vi "sirah.vi"(5 "lower limit":dbl=720.0 format="%#_13g", 6 "resonator_motor, f(x)":string="-2.10126553E+01 * x^2  + 6.31242686E+03 * x + 6.95582109E+05", 7 "upper limit":dbl=690.0 format="%#_13g", 8 "error in (no error)":errorcluster, 10 "wavelength (nm)":dbl=711.0001 format="%#_16g") -> (0 "error out":errorcluster, 1 "fundamental (nm)":dbl=708.9981708820242 format="%.4f", 2 "value out":dbl=711.0001 format="%#_16p")   [LabVIEW 2017]
uses:
  hardware/sirah/sirah.lvlib
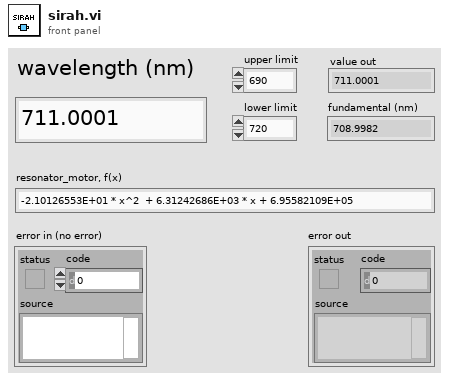
[diagram p1: front panel]
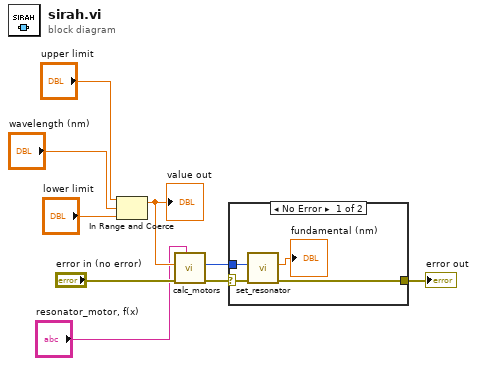
[diagram p0: block diagram]
diagram:
  n1 = In Range and Coerce(upper limit="upper limit", x="wavelength (nm)", lower limit="lower limit") -> (coerced(x)=w2:dbl)  [unwired: 1 out]
  "value out" <- w2
  n2 = call "calc_motors.vi"("resonator_motor, f(x)"="resonator_motor, f(x)", "error in (no error)"="error in (no error)", "wavelength (nm)"=w2) -> ("error out"=w7:errorcluster, "resonator"=w6:i32)  [unwired: 7 in]
  n3 = case shown="No Error" w7 {
    selector: w7 -> [w13 w14]
    tunnel: [w12 w14] -> w9
    tunnel: w6 -> [w11 _]
    frame No Error {
      n4 = call "set_resonator.vi"("error in (no error)"=w13, "resonator"=w11) -> ("error out"=w12:errorcluster, "fundamental (nm)"=→"fundamental (nm)":dbl)  [unwired: 8 in]
    }
    frame Error {
    }
  }
  "error out" <- w9
